vi "Write Setup.vi"(8 "error in":errorcluster, 10 "Setup Data":T1={"DataBase Data"={"Api Token"="", "Organization"="", "url"="", "Organization ID"=""}, "Query - csv"="", "Bucket"="", "Measurement"="", "Timestamp precision"=enum."Milliseconds", "Tags"=[{"Key"="host1", "Value"="myPC"}, {"Key"="host2", "Value"="X-Server"}]}, 11 "File Path":path) -> (0 "error out":errorcluster)   [LabVIEW 2020]
doc: "Writes all settings from the test application to the setup file"
uses:
  Setup Data.ctl
  InfluxDB v2 Client/Client/DataBase Data.ctl
  InfluxDB v2 Client/Client/Write Precision.ctl
  InfluxDB v2 Client/Data Point/Tag.ctl
  <vilib>/Utility/xml.llb/Write to XML File(string).vi
  InfluxDB v2 Client/InfluxDB v2 Client.lvlib
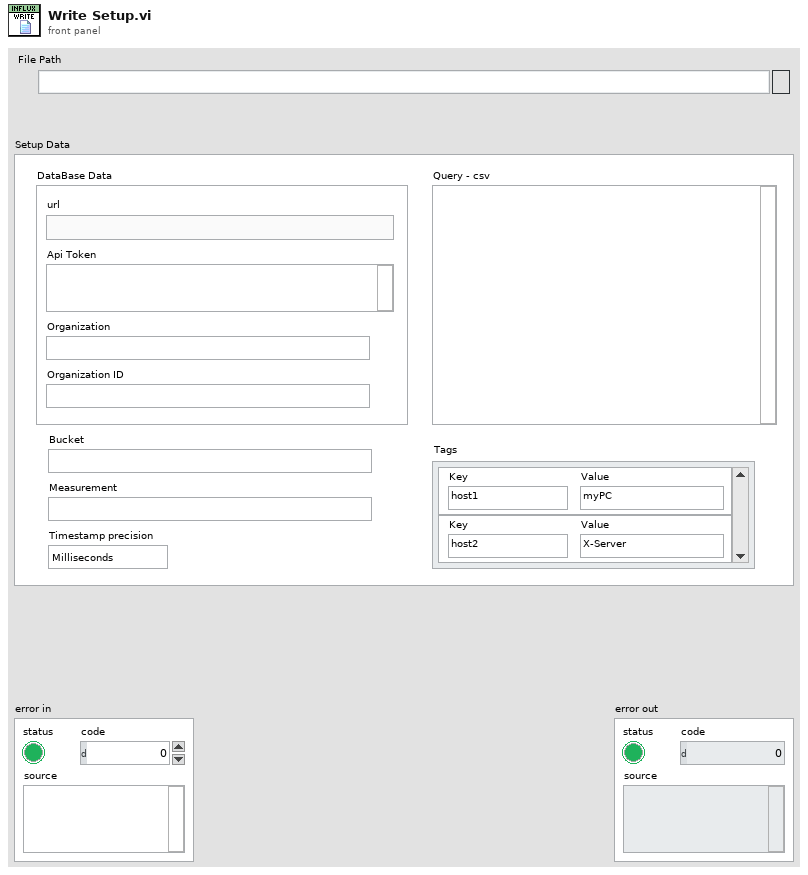
[diagram p1: front panel]
types:
  T1 = typedef "Setup Data.ctl" = cluster{"DataBase Data":T2, "Query - csv":string, "Bucket":string, "Measurement":string, "Timestamp precision":T3, "Tags":T4[]}
  T2 = typedef "InfluxDB v2 Client.lvlib/DataBase Data.ctl" = cluster{"Api Token":string, "Organization":string, "url":string, "Organization ID":string}
  T3 = typedef "InfluxDB v2 Client.lvlib/Write Precision.ctl" = enum16{"Nanoseconds", "Microseconds", "Milliseconds", "Seconds"}
  T4 = typedef "InfluxDB v2 Client.lvlib/Tag.ctl" = cluster{"Key":string, "Value":string}
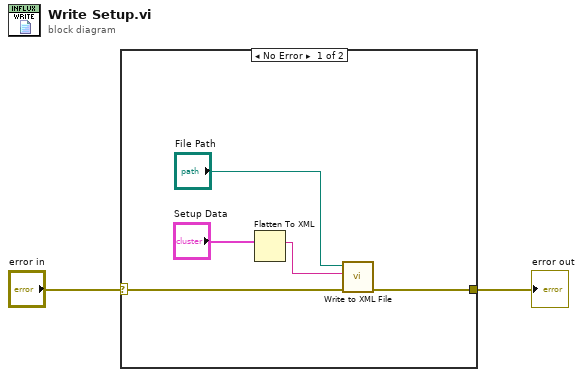
[diagram p0: block diagram]
diagram:
  n1 = case shown="No Error" "error in" {
    selector: "error in" -> [w6 w8]
    tunnel: [w3 w8] -> w1
    frame No Error {
      n2 = Flatten To XML(6:"Setup Data") -> (2:w5:string)
      n3 = call-poly <vilib>:"Write to XML File.vi"("error in (no error)"=w6, "XML Input"=w5, "XML File Path"="File Path") -> ("error out"=w3:errorcluster)  [unwired: 6 in, 2 out]
    }
    frame Error {
    }
  }
  "error out" <- w1
